vi "without_feedback.vi"() -> ()   [LabVIEW 2017]
panel:
  in  "stop":bool
  out "Avarage":dbl
  out "Random Number":dbl
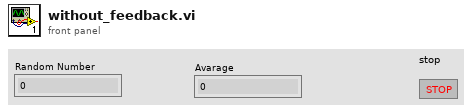
[diagram p1: front panel]
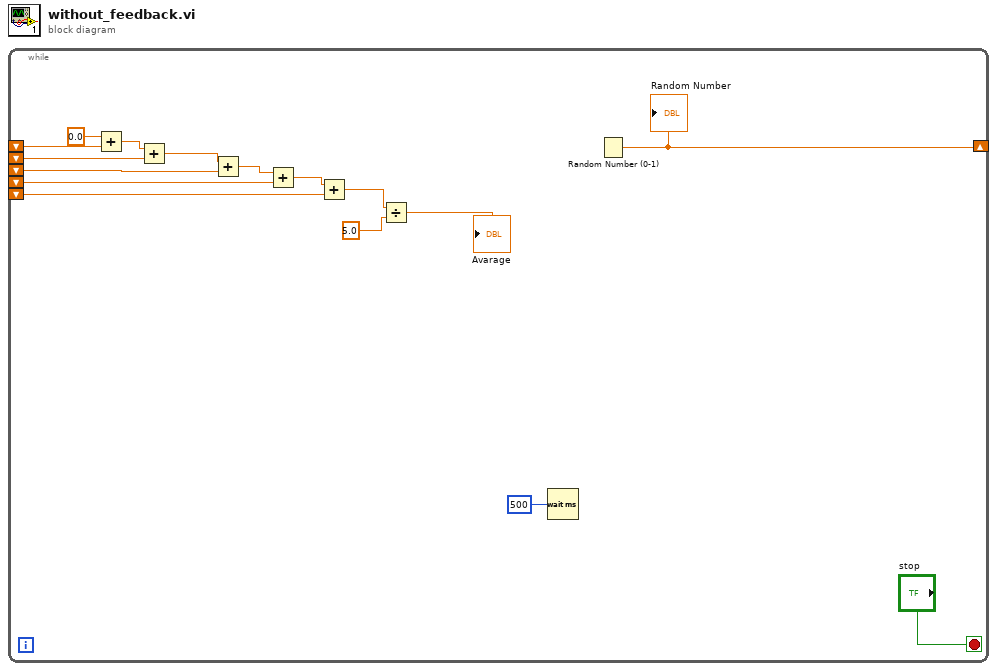
[diagram p0: block diagram]
diagram:
  n1 = while {
    shift-right: [w12] -> _
    shift-left: _ -> [w13]
    shift-left: _ -> [w11]
    shift-left: _ -> [w9]
    shift-left: _ -> [w7]
    shift-left: _ -> [w5]
    stop <- "stop" stop-if-true
    n2 = Add(x=0.0, y=w13) -> (x+y=w10:dbl)
    n3 = Add(x=w10, y=w11) -> (x+y=w8:dbl)
    n4 = Add(x=w8, y=w9) -> (x+y=w6:dbl)
    n5 = Add(x=w6, y=w7) -> (x+y=w4:dbl)
    n6 = Add(x=w4, y=w5) -> (x+y=w3:dbl)
    n7 = Divide(x=w3, y=5.0) -> (x/y=→"Avarage":dbl)
    n8 = Wait (ms)(milliseconds to wait=u32 500 ("millisecond timer value")) -> ()  [unwired: 1 out]
    n9 = Random Number (0-1)() -> (number: 0 to 1=w12:dbl)
    "Random Number" <- w12
  }
